vi "GenEdgeTrigger.vi"() -> ()   [LabVIEW 2020]
doc: "Calculate rate for general purpose\n Inputs: time in seconds, and distnce in units\nCalculates rate value (Distance/time(s))"
panel:
  out "Prior State":bool
  out "?":bool
  in  "Current State":bool
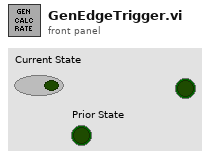
[diagram p1: front panel]
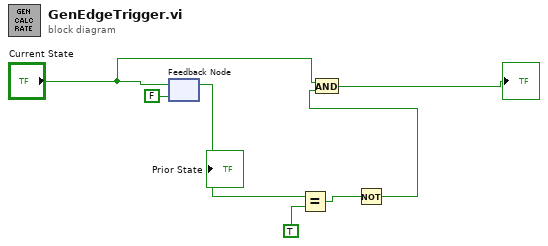
[diagram p0: block diagram]
diagram:
  n1 = feedback #1(FALSE ("Current State")) -> (w4:bool)
  "Prior State" <- w4
  n2 = feedback-in #1("Current State") -> ()
  n3 = Equal?(x=w4, y=TRUE) -> (x = y?=w6:bool)
  n4 = Not(x=w6) -> (.not. x?=w2:bool)
  n5 = And(x="Current State", y=w2) -> (x .and. y?=→"?":bool)
